vi "UploadFile.vi"(7 "Root Path":path, 8 "error in (no error)":errorcluster, 10 "Path":path, 11 "Protocol in":refnum<class "Protocol.lvclass">) -> (0 "error out":errorcluster, 3 "Protocol out":refnum<class "Protocol.lvclass">)   [LabVIEW 2020, in "FileSync -- Base.lvlib" / "Protocol.lvclass"]
uses:
  Protocol.lvclass
  Protocol.lvclass/Protocol.ctl
  <vilib>/NI/Tools/String/Tools_String.lvlib
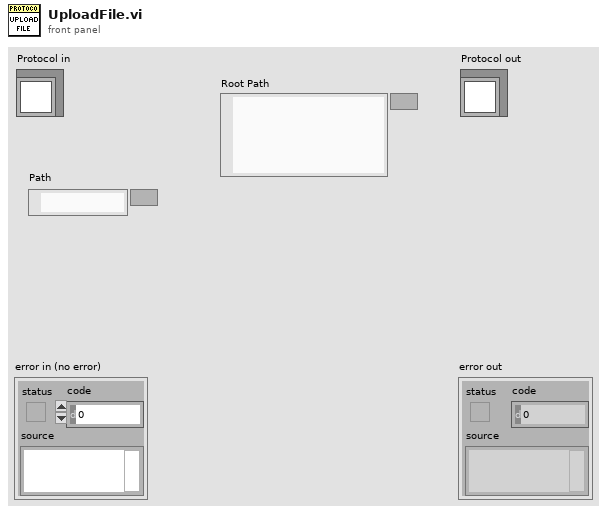
[diagram p1: front panel]
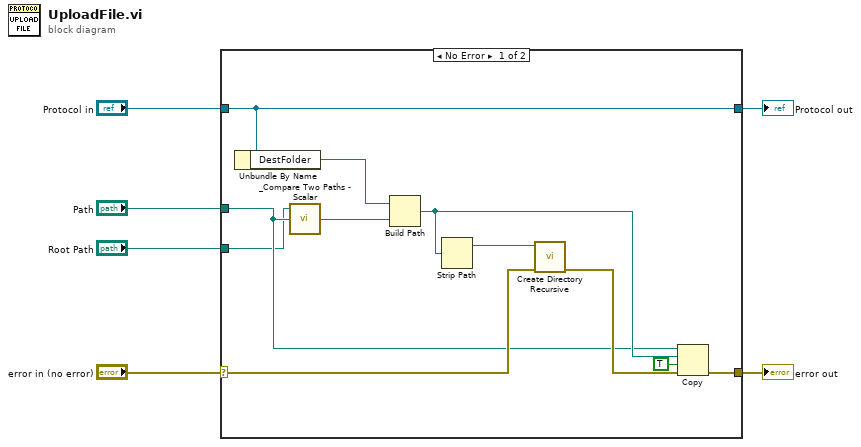
[diagram p0: block diagram]
diagram:
  n1 = case shown="No Error" "error in (no error)" {
    selector: "error in (no error)" -> [w17 w19]
    tunnel: [w13 w19] -> w5
    tunnel: [w16 w18] -> w3
    tunnel: "Protocol in" -> [w16 w18]
    tunnel: "Path" -> [w9 _]
    tunnel: "Root Path" -> [w8 _]
    frame No Error {
      n2 = Unbundle By Name(w16) -> ("DestFolder"=w15:path)
      n3 = call "_Compare Two Paths - Scalar.vi"("path2"=w9, "path1"=w8) -> ("relative path from 1 to 2"=w14:path)  [unwired: 1 in, 2 out]
      n4 = Build Path(base path=w15, name or relative path=w14) -> (appended path=w12:path)
      n5 = Strip Path(path=w12) -> (stripped path=w10:path)  [unwired: 1 out]
      n6 = call <vilib>:"Create Directory Recursive.vi"("error in"=w17, "directory"=w10) -> ("error out"=w11:errorcluster)  [unwired: 4 in, 1 out]
      n7 = Copy(8:w11, 9:TRUE ("overwrite (F)"), 10:w12, 11:w9) -> (0:w13:errorcluster)  [unwired: 1 in, 2 out]
    }
    frame Error {
    }
  }
  "error out" <- w5
  "Protocol out" <- w3
